vi "JV_curve.vi"(0 "Start (V)":sgl=1.2, 1 "End (V)":sgl=-0.2, 2 "vs init":bool[](array[boolean])=[FALSE, FALSE], 3 "Equilibration time (s)":sgl=1.0 min=0 max=1000, 4 "Equilibration time back (s)":sgl min=0 max=1000, 5 "error in (no error)":errorcluster, 6 "Device Code":i32=16, 7 "Hysteresis":bool=TRUE, 8 "instance":i32, 9 "VoltageRange abs and vs init":dbl[][](array[numeric])=[[-1.0, -2.0], [1.5, 0.2]], 10 "ID":i32=6, 11 "Record every dE (mV)":sgl=100.0, 12 "Channel":u8(ring) items=["1", "2", "3", "4", "5", "6", "7", "8", "9", "10", "11", "12", "13", "14", "15", "16"], 13 "Scan rate (mV/s)":sgl=300.0, 17 "Device Area cm2":sgl=0.16) -> (14 "JVData":sgl[][](array[numeric]) format="%.2f", 15 "JVParameters1st":dbl[](array[numeric])=[nan, nan, nan, -0.0, 0.0, -0.0], 16 "In range?":bool=TRUE, 18 "JVParameters2nd":dbl[](array[numeric])=[nan, nan, nan, -0.0, 0.0, -0.0], 19 "error out":errorcluster={"status"=TRUE, "code"=-1, "source"="DLL"})   [LabVIEW 2020]
uses:
  base_xml.llb/Type Descriptor Enumeration__ogtk.ctl
  ActiveArray.vi
panel:
  out "AverageVoc":dbl=nan
  out "IVData":sgl[][](array[numeric]) format="%.2f"
  out "finished":bool=TRUE
  out "Exit 2":bool
  out "Number of\nJV points":i32
  in  "JV measurement":enum16{"I(Ewe)", "Ewe(t)", "I(t)", "P(Ewe)"}(ring) caption="Draw"
  out "XY Graph":cluster{"JVData":sgl[], "JVData":sgl[]}(graph)
  in  "stop":bool
  in  "VSCAN Parameters":T1={"tb"=0.00025, "vs_initial "=FALSE, "Voltage_step"=1.2, "Scans"=[{" vs_initial "=FALSE, "Voltage_step"=-0.2, "Scan_Rate"=1.0}, {" vs_initial "=FALSE, "Voltage_step"=-0.2, "Scan_Rate"=1.0}, {" vs_initial "=FALSE, "Voltage_step"=-0.2, "Scan_Rate"=1.0}, {" vs_initial "=FALSE, "Voltage_step"=-0.2, "Scan_Rate"=1.0}, {" vs_initial "=FALSE, "Voltage_step"=-0.2, "Scan_Rate"=1.0}, {" vs_initial "=FALSE, "Voltage_step"=-0.2, "Scan_Rate"=1.0}], "Scan_number"=3, "N_Cycles"=0, "Record_every_dE"=0.1, "Begin_measuring_I"=0.5, "End_measuring_I"=0.75, "I_Range"=12, "E_Range"=3, "Bandwidth"=5, "em"=0, "ce"=0} {"tb" min=5e-05 max=1 format="%^_3e"; "ce" items=["Standard", "CE to ground"]; "End_measuring_I" min=0 max=1 format="%.2f"; "Begin_measuring_I" min=0 max=1 format="%.2f"; "Voltage_step" min=-10 max=10 format="%^_3e"; "N_Cycles" min=0 max=1000000; "Scan_number" min=0 max=98; "Scans"."Scan_Rate" min=1e-05 max=10 format="%^_3e"; "Scans"."Voltage_step" format="%^_3e"; "E_Range" items=["±2.5V", "±5V", "±10V", "Auto"]; "Bandwidth" items=["1"=1, "2"=2, "3"=3, "4"=4, "5"=5, "6"=6, "7"=7, "8"=8, "9"=9]; "Record_every_dE" format="%^_3e"; "I_Range" items=["1pA", "1nA", "10nA", "100nA", "1µA", "10µA", "100µA", "1mA", "10mA", "100mA", "1A", "Booster", "Auto"]}
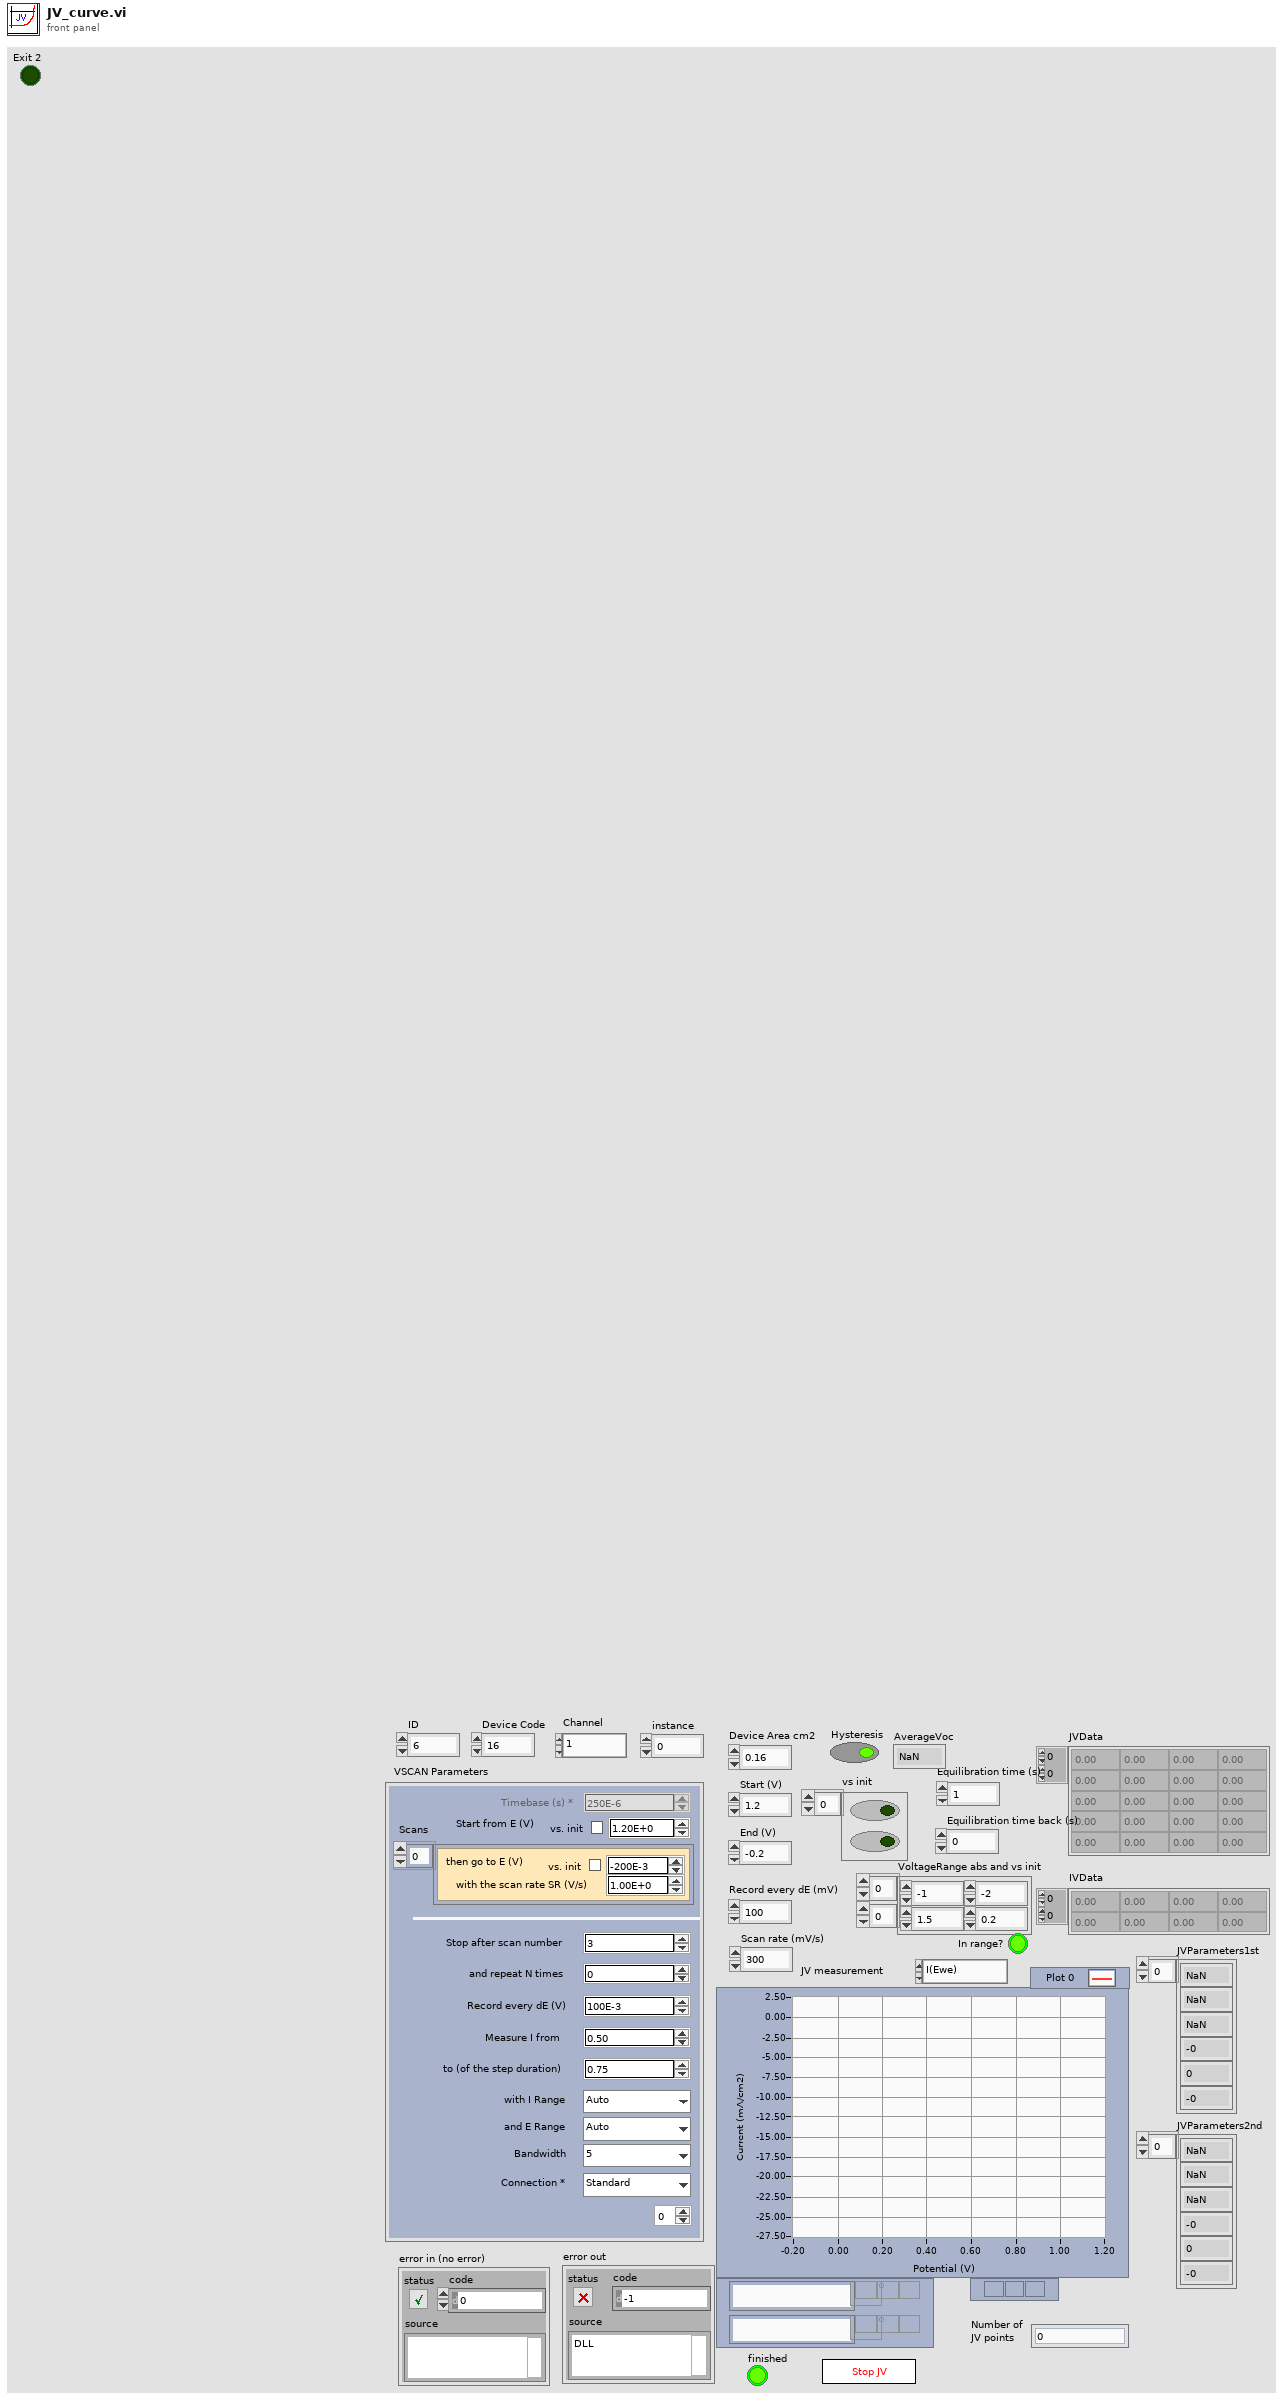
[diagram p1: front panel]
types:
  T1 = cluster{"tb":sgl, "vs_initial ":bool, "Voltage_step":sgl, "Scans":cluster{" vs_initial ":bool, "Voltage_step":sgl, "Scan_Rate":sgl}[], "Scan_number":i32, "N_Cycles":i32, "Record_every_dE":sgl, "Begin_measuring_I":sgl, "End_measuring_I":sgl, "I_Range":u16, "E_Range":u16, "Bandwidth":u16, "em":u16, "ce":u16}
  T2 = typedef "Type Descriptor Enumeration__ogtk.ctl" = enum8{"<Null>", "I8", "I16", "I32", "I64", "U8", "U16", "U32", "U64", "SGL", "DBL", "EXT", "CSG", "CDB", "CXT", "0x0F", "0x10", "0x11", "0x12", "0x13", "0x14", "Enum U8", "Enum U16", "Enum U32", "Enum U64", "SGL PQ", "DBL PQ", "EXT PQ", "CSG PQ", "CDB PQ", "CXT PQ", "0x1F", "0x20", "Boolean", "0x22", "0x23", "0x24", "0x25", "0x26", "0x27", "0x28", "0x29", "0x2A", "0x2B", "0x2C", "0x2D", "0x2E", "0x2F", "String", "0x31", "Path", "Pict", "0x34", "0x35", "0x36", "DAQ", "0x38", "0x39", "0x3A", "0x3B", "0x3C", "0x3D", "0x3E", "0x3F", "Array", "0x41", "0x42", "0x43", "0x44", "0x45", "0x46", "0x47", "0x48", "0x49", "0x4A", "0x4B", "0x4C", "0x4D", "0x4E", "0x4F", "Cluster", "0x51", "0x52", "Variant", "Waveform", "0x55", "0x56", "0x57", "0x58", "0x59", "0x5A", "0x5B", "0x5C", "0x5D", "0x5E", "0x5F", "0x60", "0x61", "0x62", "0x63", "0x64", "0x65", "0x66", "0x67", "0x68", "0x69", "0x6A", "0x6B", "0x6C", "0x6D", "0x6E", "0x6F", "Refnum"}
  T3 = cluster{"Data Type":T2, "Format String":string}[]
  T4 = cluster{" vs_initial ":bool, "Voltage_step":sgl, "Scan_Rate":sgl}[]
  T5 = cluster{" vs_initial ":bool, "Voltage_step":sgl, "Scan_Rate":sgl}
  T6 = cluster{"Label":string, "type":i32, "valeur":u32, "index":i32}[]
  T7 = cluster{"IRQskipped":i32, "NbRaws":i32, "NbCols":i32, "Technique Index":i32, "TechniqueID":i32, "PrcessIndex":i32, "loop":i32, "StartTime":dbl, "MuxPad":i32}
  T8 = cluster{"State":i32, "MemFilled":i32, "TimeBase":sgl, " Ewe":sgl, " EweRangeMin":sgl, " EweRangeMax":sgl, "Ece":sgl, "EceRangeMin":sgl, "EceRangeMax":sgl, "Eoverflow":i32, "I":sgl, "IRange":i32, "Ioverflow":i32, "ElapsedTime":sgl, "Freq":sgl, "Rcomp":sgl, "Saturation":sgl, "OptErr":i32, "OptPos":i32}
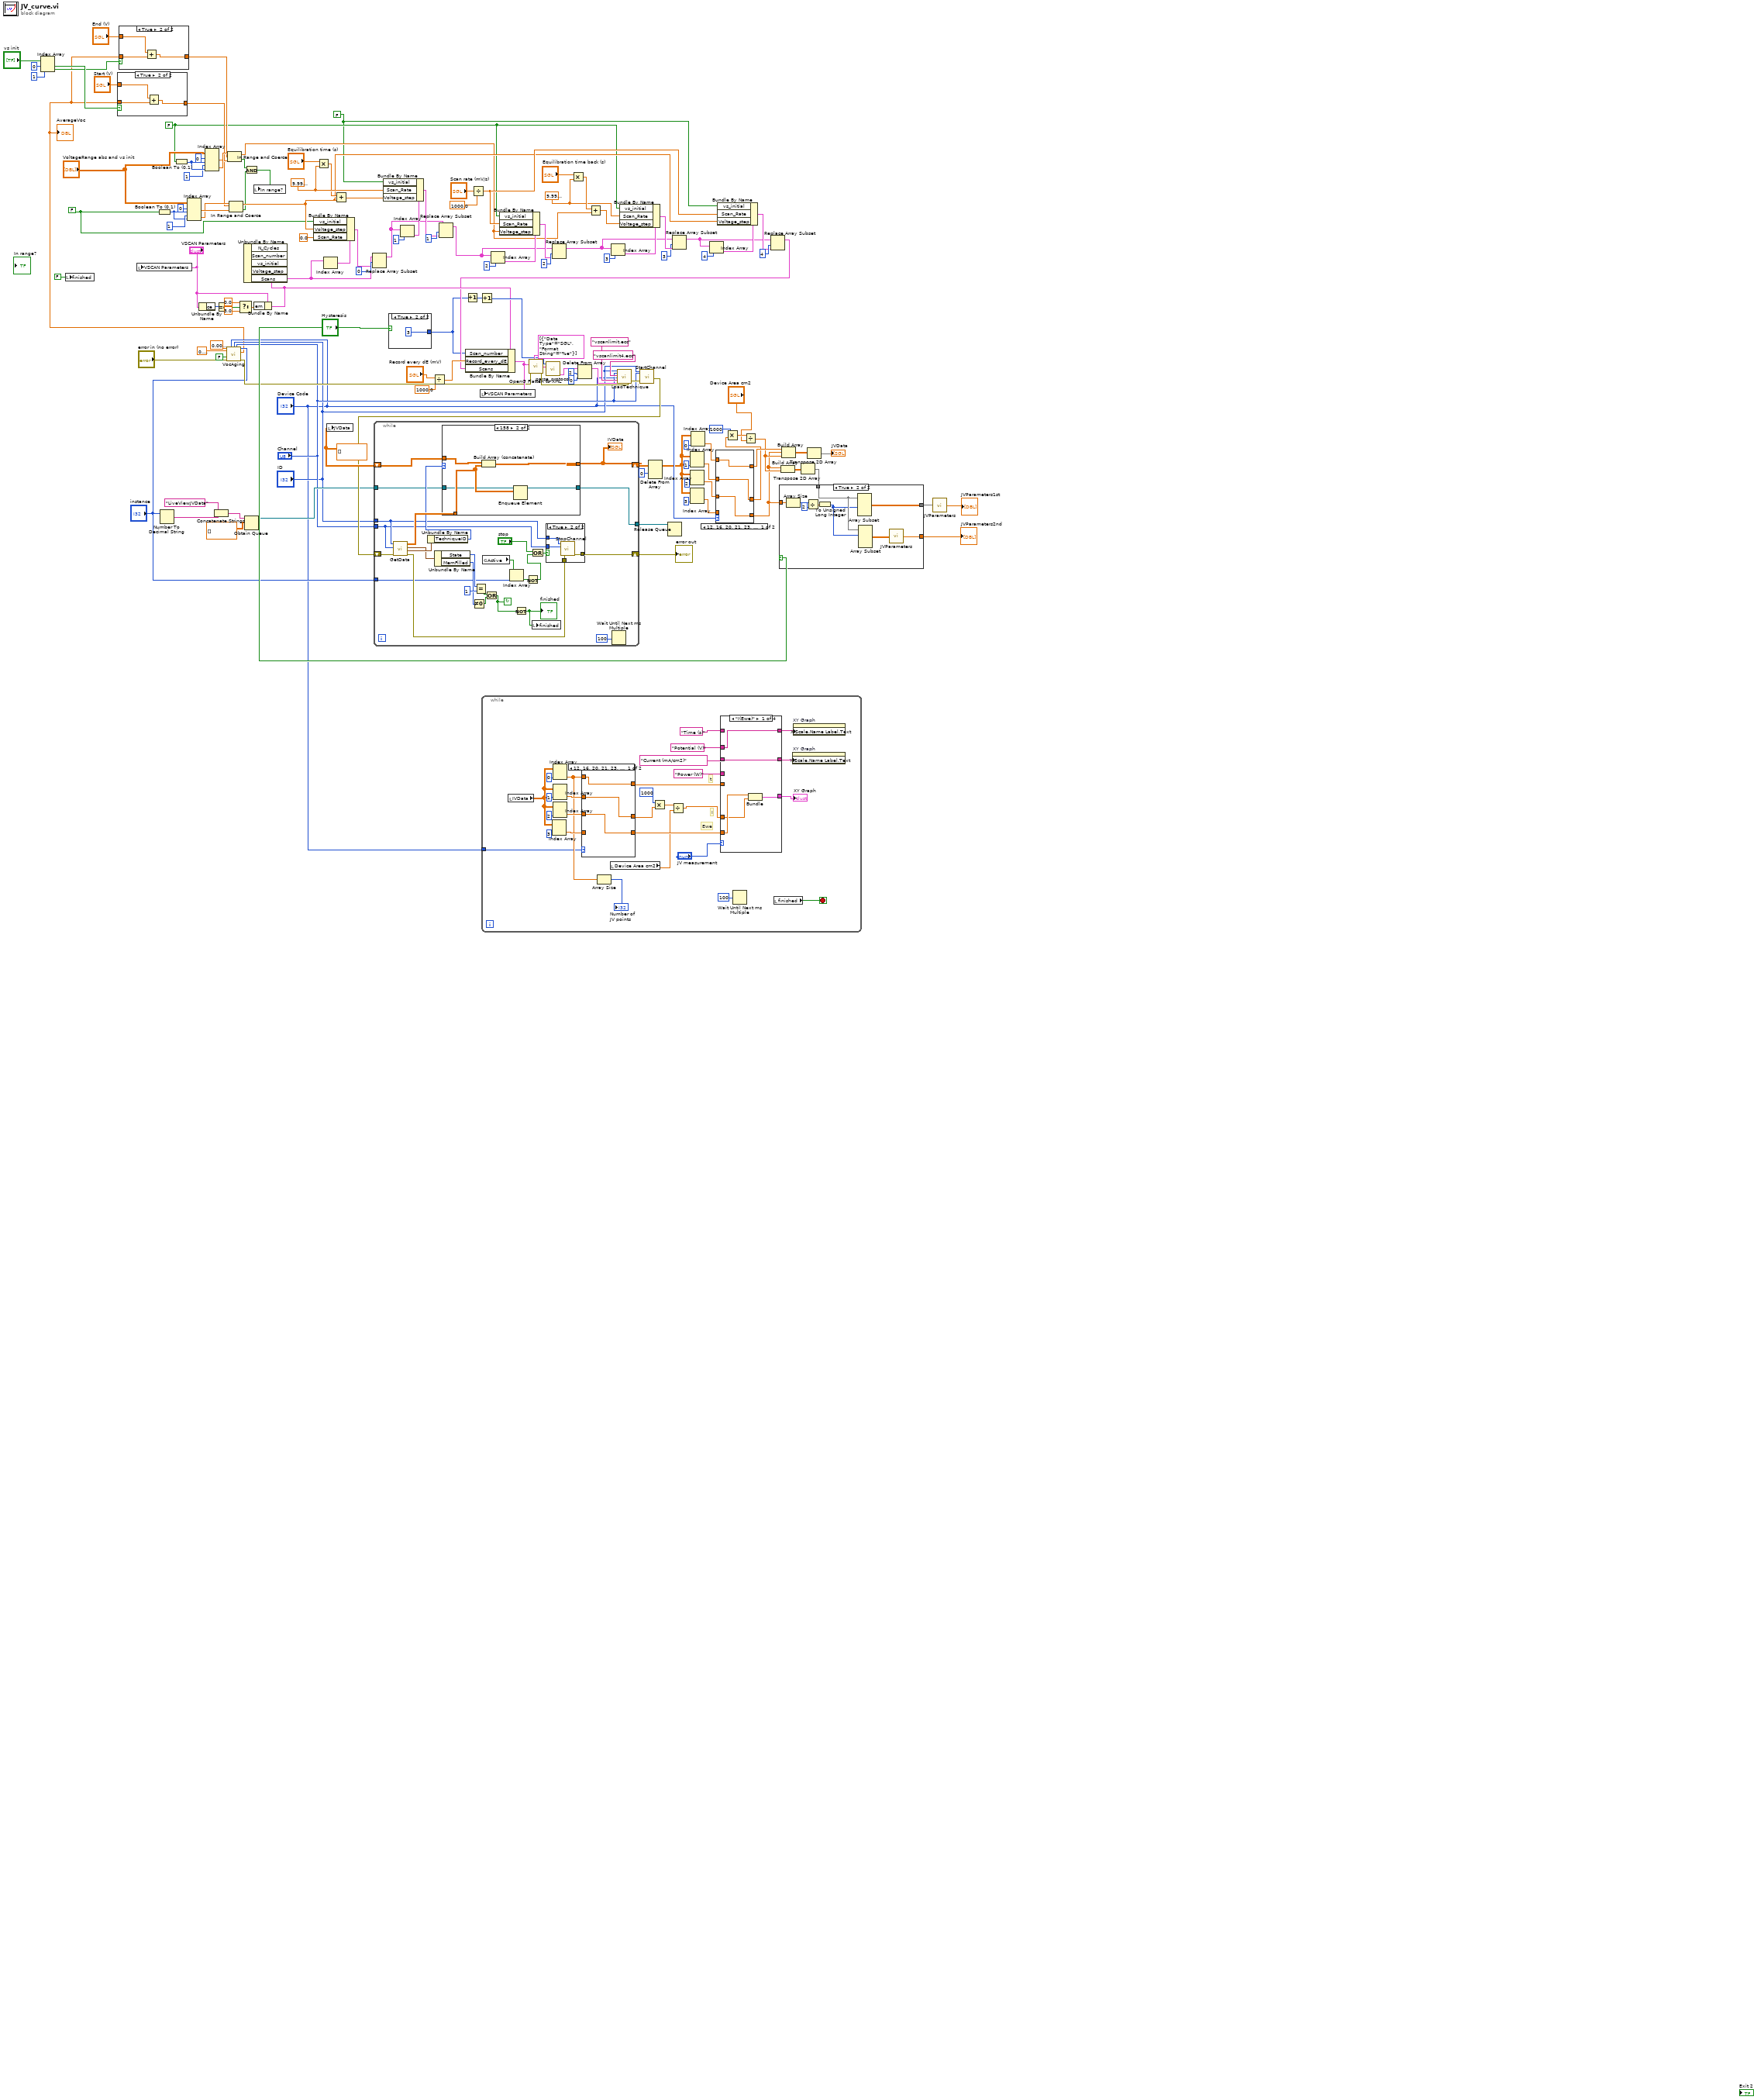
[diagram p0: block diagram]
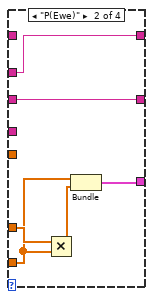
[diagram p4: hidden frame]
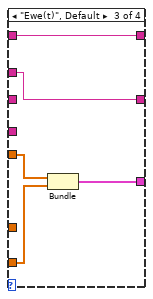
[diagram p5: hidden frame]
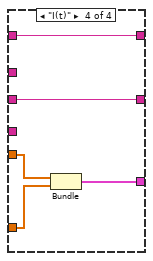
[diagram p6: hidden frame]
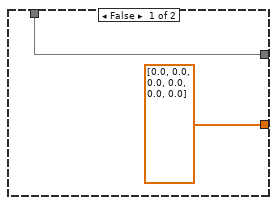
[diagram p8: hidden frame]
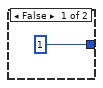
[diagram p10: hidden frame]
diagram:
  w9 = FALSE
  w10 = FALSE
  w11 = FALSE
  w82 = sgl 0.0001 ("Scan_Rate")
  w94 = sgl 0.0001 ("Scan_Rate")
  w133 = sgl[][] []
  n1 = Index Array(array="vs init", index #1=0 ("index"), index #2=1 ("index")) -> (element #1=w8:bool, element #2=w7:bool)
  n2 = local write "finished"(FALSE ("finished")) -> ()
  n3 = local write "VSCAN Parameters"("VSCAN Parameters") -> ()
  n4 = Boolean To (0,1)(Boolean=w10) -> (0, 1=w35:i16)
  n5 = Number To Decimal String(number="instance") -> (decimal integer string=w51:string)  [unwired: 1 in]
  n6 = Boolean To (0,1)(Boolean=w11) -> (0, 1=w30:i16)
  n7 = Index Array(array="VoltageRange abs and vs init", index (row) #1=0 ("disabled index (row)"), index (col) #1=w35, index (row) #2=1 ("length"), index (col) #2=w35) -> (element #1=w34:dbl, element #2=w33:dbl)
  n8 = Unbundle By Name("VSCAN Parameters") -> ("ce"=w116:u16)
  n9 = Index Array(array="VoltageRange abs and vs init", index (row) #1=0 ("disabled index (row)"), index (col) #1=w30, index (row) #2=1 ("length"), index (col) #2=w30) -> (element #1=w31:dbl, element #2=w32:dbl)
  n10 = Concatenate Strings("LiveViewJVData" ("name (unnamed)"), w51) -> (w52:string)
  n11 = Equal To 0?(x=w116) -> (x = 0?=w115:bool)
  n12 = call "VocAging.vi"("time at OC (min)"=sgl 0.01, "Device Code"="Device Code", "ID"="ID", "Channel"="Channel", "instance"="instance", "Record_every_dT (s)"=sgl 0.1, "Save Data"=FALSE, "error in (no error)"="error in (no error)") -> ("AverageVoc"=w4:dbl, "error out"=w20:errorcluster)  [unwired: 6 in]
  "AverageVoc" <- w4
  n13 = case shown="True" w8 {
    tunnel: [w136 w138] -> w12
    tunnel: "Start (V)" -> [w136 w139]
    tunnel: w4 -> [_ w137]
    frame False {
    }
    frame True {
      n14 = Add(x=w139, y=w137) -> (x+y=w138:dbl)
    }
  }
  n15 = case shown="True" w7 {
    tunnel: [w140 w141] -> w26
    tunnel: "End (V)" -> [w140 w143]
    tunnel: w4 -> [_ w142]
    frame False {
    }
    frame True {
      n16 = Add(x=w143, y=w142) -> (x+y=w141:dbl)
    }
  }
  n17 = In Range and Coerce(upper limit=w32, x=w26, lower limit=w31) -> (coerced(x)=w25:dbl, In Range?=w24:bool)
  n18 = In Range and Coerce(upper limit=w33, x=w12, lower limit=w34) -> (coerced(x)=w38:dbl, In Range?=w23:bool)
  n19 = Select(t=0.0, s=w115, f=3.0) -> (s? t:f=w118:dbl)
  n20 = Obtain Queue(name (unnamed)=w52, element data type=sgl[][] []) -> (queue out=w49:refnum<queue>)  [unwired: 3 in, 2 out]
  n21 = And(x=w24, y=w23) -> (x .and. y?=w22:bool)
  n22 = local write "In range?"(w22) -> ()
  n23 = Bundle By Name(cluster="VSCAN Parameters", "em"=w118) -> (w114:T1)
  n24 = Unbundle By Name(w114) -> ("Scans"=w110:T4)  [unwired: 4 out]
  n25 = Multiply(x="Equilibration time (s)", y=w94) -> (x*y=w92:sgl)
  n26 = Index Array(array=w110) -> (element=w122:T5)  [unwired: 1 in]
  n27 = Bundle By Name(cluster=w122, "vs_initial"=w10, "Voltage_step"=w38, "Scan_Rate"=sgl 0.0) -> (w124:T5)
  n28 = local write "JVData"(w133) -> ()
  n29 = Add(x=w92, y=w38) -> (x+y=w91:dbl)
  n30 = Replace Array Subset(array=w110, new element=w124, index=0 ("indice")) -> (w95:T4)
  n31 = case shown="True" "Hysteresis" {
    tunnel: [1 ("index") 3 ("index")] -> w72
    frame False {
    }
    frame True {
    }
  }
  n32 = Index Array(array=w95, index=1) -> (element=w96:T5)
  n33 = Bundle By Name(cluster=w96, "vs_initial"=w9, "Scan_Rate"=w94, "Voltage_step"=w91) -> (w98:T5)
  n34 = Divide(x="Record every dE (mV)", y=sgl 1000.0) -> (x/y=w103:sgl)
  n35 = Replace Array Subset(array=w95, new element=w98, index=1 ("indice")) -> (w90:T4)
  n36 = Increment(x=w72) -> (x+1=w121:i32)
  n37 = Divide(x="Scan rate (mV/s)", y=sgl 1000.0) -> (x/y=w75:sgl)
  n38 = Increment(x=w121) -> (x+1=w120:i32)
  n39 = while {
    tunnel: "Device Code" -> [w146]
    stop <- w172 stop-if-true
    # "Ewe"
    # "I"
    # "t"
    n40 = local read "IVData"() -> (w163:sgl[][])
    n41 = Index Array(array=w163, index (col)=3 ("Index")) -> (element=w165:sgl[])  [unwired: 1 in]
    n42 = Index Array(array=w163, index (col)=1 ("Index")) -> (element=w168:sgl[])  [unwired: 1 in]
    n43 = Index Array(array=w163, index (col)=2 ("Index")) -> (element=w166:sgl[])  [unwired: 1 in]
    n44 = Index Array(array=w163, index (col)=0 ("Index")) -> (element=w162:sgl[])  [unwired: 1 in]
    n45 = case shown="12, 16, 20, 21, 23, 27" w146 {
      tunnel: w168 -> [w196 _]
      tunnel: w166 -> [w195 w199]
      tunnel: w165 -> [_ w198]
      tunnel: w162 -> [w197 w200]
      tunnel: [w197 w200] -> w154
      tunnel: [w196 w199] -> w148
      tunnel: [w195 w198] -> w153
      frame 12, 16, 20, 21, 23, 27 {
      }
      frame Default {
      }
    }
    n46 = Array Size(array=w162) -> (size(s)=→"Number of\nJV points":i32)
    n47 = local read "Device Area cm2"() -> (w149:sgl)
    n48 = Multiply(x=1000, y=w148) -> (x*y=w151:sgl[])
    n49 = Divide(x=w151, y=w149) -> (x/y=w150:sgl[])
    n50 = case shown="\"I(Ewe)\"" "JV measurement" {
      tunnel: w154 -> [_ _ w189 w194]
      tunnel: w150 -> [w175 w181 _ w193]
      tunnel: [w174 w182 w185 w190] -> w161
      tunnel: "Potential (V)" ("Y Scale.Name Label.Text") -> [w178 w184 w188 _]
      tunnel: "Current (mA/cm2)" ("Y Scale.Name Label.Text") -> [w177 w183 _ w192]
      tunnel: [w177 w183 w188 w192] -> w159
      tunnel: [w178 w184 w187 w191] -> w158
      tunnel: "Time (s)" ("Y Scale.Name Label.Text") -> [_ _ w187 w191]
      tunnel: w153 -> [w176 w180 w186 _]
      tunnel: "Power (W)" ("Y Scale.Name Label.Text") -> [_ _ _ _]
      frame "I(Ewe)" {
        n51 = Bundle("IVData"=w176, w175) -> (w174:cluster{"IVData":sgl[], sgl[]})  [unwired: 1 in]
      }
      frame "P(Ewe)" {
        n52 = Multiply(x=w181, y=w180) -> (x*y=w179:sgl[])
        n53 = Bundle("IVData"=w180, w179) -> (w182:cluster{"IVData":sgl[], sgl[]})  [unwired: 1 in]
      }
      frame "Ewe(t)", Default {
        n54 = Bundle("IVData"=w189, "IVData"=w186) -> (w185:cluster{"IVData":sgl[], "IVData":sgl[]})  [unwired: 1 in]
      }
      frame "I(t)" {
        n55 = Bundle("IVData"=w194, w193) -> (w190:cluster{"IVData":sgl[], sgl[]})  [unwired: 1 in]
      }
    }
    "XY Graph" <- w161
    n56 = Wait Until Next ms Multiple(millisecond multiple=u32 100) -> ()  [unwired: 1 out]
    n57 = local read "finished"() -> (w172:bool)
    n58 = property on="XY Graph" class="XYGraph (strict)"("Y Scale.Name Label.Text"=w159) -> ()  [unwired: 2 in, 2 out]
    n59 = property on="XY Graph" class="XYGraph (strict)"("X Scale.Name Label.Text"=w158) -> ()  [unwired: 2 in, 2 out]
  }
  n60 = Index Array(array=w90, index=2) -> (element=w108:T5)
  n61 = Bundle By Name(cluster=w108, "vs_initial"=w11, "Scan_Rate"=w75, "Voltage_step"=w25) -> (w111:T5)
  n62 = Replace Array Subset(array=w90, new element=w111, index=2 ("indice")) -> (w85:T4)
  n63 = Multiply(x="Equilibration time back (s)", y=w82) -> (x*y=w84:sgl)
  n64 = Add(x=w84, y=w25) -> (x+y=w81:dbl)
  n65 = Index Array(array=w85, index=3) -> (element=w89:T5)
  n66 = Bundle By Name(cluster=w89, "vs_initial"=w11, "Scan_Rate"=w82, "Voltage_step"=w81) -> (w87:T5)
  n67 = Replace Array Subset(array=w85, new element=w87, index=3 ("indice")) -> (w76:T4)
  n68 = Index Array(array=w76, index=4) -> (element=w77:T5)
  n69 = Bundle By Name(cluster=w77, "vs_initial"=w9, "Scan_Rate"=w75, "Voltage_step"=w38) -> (w79:T5)
  n70 = Replace Array Subset(array=w76, new element=w79, index=4 ("indice")) -> (w74:T4)
  n71 = Bundle By Name(cluster=w114, "Scan_number"=w72, "Record_every_dE"=w103, "Scans"=w74) -> (w104:T1)
  n72 = local write "VSCAN Parameters"(w104) -> ()
  n73 = call "OpenG Flatten to XML.vi"("Type Formats (default)"=T3 [{"Data Type"=enum."SGL", "Format String"="%e"}] ("Type Formats"), "error in (no error)"=w20, "LabVIEW Data"=w104) -> ("error out"=w130:errorcluster, "XML String"=w131:string)  [unwired: 7 in]
  n74 = call "parse_protocol.vi"("XML String In"=w131, "index array"=w120) -> ("Params Values"=w127:T6)  [unwired: 7 in]
  n75 = Delete From Array(array=w127, length=2 ("longueur"), index=0 ("indice")) -> (array with subset deleted=w126:T6)  [unwired: 1 out]
  n76 = call "LoadTechnique.vi"("ID"="ID", "Selected Channel"="Channel", "FName4"="vscanlimit4.ecc" ("FName"), "Device Code"="Device Code", "FName"="vscanlimit.ecc", "Protocol Parameters"=w126, "error in (no error)"=w130) -> ("error out"=w134:errorcluster)  [unwired: 12 in]
  n77 = call "StartChannel.vi"("error in (no error)"=w134, "Channel"="Channel", "ID"="ID") -> ("error out"=w100:errorcluster)  [unwired: 8 in]
  n78 = while {
    shift-right: [w221] -> w73
    shift-left: w100 -> [w223]
    shift-right: [w203] -> w3
    shift-left: w133 -> [w219]
    tunnel: "Channel" -> [w201]
    tunnel: "ID" -> [w216]
    tunnel: w49 -> [w205]
    tunnel: [w204] -> w48
    tunnel: "instance" -> [w202]
    stop <- w211 continue-if-true
    n79 = call "GetData.vi"("error in (no error)"=w223, "Channel"=w201, "ID"=w216) -> ("error out"=w218:errorcluster, "Data information"=w227:T7, "Current values"=w215:T8, "Data"=w220:dbl[][])  [unwired: 5 in]
    n80 = Unbundle By Name(w227) -> ("TechniqueID"=w217:i32)
    n81 = Unbundle By Name(w215) -> ("State"=w214:i32, "MemFilled"=w213:i32)
    n82 = case shown="158" w217 {
      tunnel: w220 -> [_ w239]
      tunnel: w219 -> [w234 w238]
      tunnel: [w234 w237] -> w203
      tunnel: w205 -> [w233 w236]
      tunnel: [w233 w235] -> w204
      frame 0, Default {
      }
      frame 158 {
        n83 = Build Array (concatenate)(w238, w239) -> (w237:dbl[][])
        n84 = Enqueue Element(queue=w236, element=w239) -> (queue out=w235:refnum<queue>)  [unwired: 2 in, 2 out]
      }
    }
    "IVData" <- w203
    n85 = Not Equal To 0?(x=w213) -> (x != 0?=w224:bool)
    n86 = Equal?(x=w214, y=1) -> (x = y?=w225:bool)
    n87 = global read "ActiveArray.vi" "Active"() -> (w210:bool[])
    n88 = Or(x=w225, y=w224) -> (x .or. y?=w211:bool)
    n89 = Index Array(array=w210, index=w202) -> (element=w209:bool)
    n90 = Not(x=w211) -> (.not. x?=w212:bool)
    "finished" <- w212
    n91 = Not(x=w209) -> (.not. x?=w206:bool)
    n92 = Or(x="stop", y=w206) -> (x .or. y?=w208:bool)
    n93 = local write "finished"(w212) -> ()
    n94 = case shown="True" w208 {
      tunnel: [w228 w232] -> w221
      tunnel: w218 -> [w228 w231]
      tunnel: w201 -> [_ w230]
      tunnel: w216 -> [_ w229]
      frame False {
      }
      frame True {
        n95 = call "StopChannel.vi"("error in (no error)"=w231, "Channel"=w230, "ID"=w229) -> ("error out"=w232:errorcluster)  [unwired: 8 in]
      }
    }
    n96 = Wait Until Next ms Multiple(millisecond multiple=u32 100) -> ()  [unwired: 1 out]
  }
  "error out" <- w73
  n97 = Delete From Array(array=w3, index (row)=0) -> (array with subset deleted=w2:dbl[][])  [unwired: 2 in, 1 out]
  n98 = Release Queue(queue=w48) -> ()  [unwired: 2 in, 3 out]
  n99 = Index Array(array=w2, index (col)=3 ("Index")) -> (element=w65:dbl[])  [unwired: 1 in]
  n100 = Index Array(array=w2, index (col)=1 ("Index")) -> (element=w68:dbl[])  [unwired: 1 in]
  n101 = Index Array(array=w2, index (col)=2 ("Index")) -> (element=w66:dbl[])  [unwired: 1 in]
  n102 = Index Array(array=w2, index (col)=0 ("Index")) -> (element=w64:dbl[])  [unwired: 1 in]
  n103 = case shown="12, 16, 20, 21, 23, 27" "Device Code" {
    tunnel: w68 -> [w241 _]
    tunnel: w66 -> [w240 w244]
    tunnel: w65 -> [_ w243]
    tunnel: w64 -> [w242 w245]
    tunnel: [w242 w245] -> w47
    tunnel: [w241 w244] -> w46
    tunnel: [w240 w243] -> w42
    frame 12, 16, 20, 21, 23, 27 {
    }
    frame Default {
    }
  }
  n104 = Multiply(x=1000, y=w46) -> (x*y=w62:dbl[])
  n105 = Divide(x=w62, y="Device Area cm2") -> (x/y=w45:dbl[])
  n106 = Build Array(w42, w45) -> (w61:dbl[][])
  n107 = Build Array(w47, w42, w45) -> (w44:dbl[][])
  n108 = Transpose 2D Array(2D array=w61) -> (transposed array=w60:dbl[][])
  n109 = case shown="True" "Hysteresis" {
    tunnel: w42 -> [_ w256]
    tunnel: w60 -> [w247 w251]
    tunnel: [w247 w252] -> w58
    tunnel: [dbl[] [0.0, 0.0, 0.0, 0.0, 0.0, 0.0] ("JVParameters") w248] -> w56
    frame False {
    }
    frame True {
      n110 = Array Size(array=w256) -> (size(s)=w255:i32)
      n111 = Divide(x=w255, y=2) -> (x/y=w253:dbl)
      n112 = To Unsigned Long Integer(number=w253) -> (unsigned 32bit integer=w250:u32)
      n113 = Array Subset(array=w251, length (row)=w250) -> (w252:dbl[][])  [unwired: 3 in]
      n114 = Array Subset(array=w251, index (row)=w250) -> (w249:dbl[][])  [unwired: 3 in]
      n115 = call "JVParameters.vi"("InputJV"=w249) -> ("JVParameters"=w248:dbl[])
    }
  }
  "JVParameters2nd" <- w56
  n116 = Transpose 2D Array(2D array=w44) -> (transposed array=→"JVData":dbl[][])
  n117 = call "JVParameters.vi"("InputJV"=w58) -> ("JVParameters"=→"JVParameters1st":dbl[])
